vi "Temperature Limit.vi"() -> ()   [LabVIEW 2015]
doc: "This VI simulates the acquisition of temperature, graphs the temperature, and notifies the user if the temperature is over the limit."
panel:
  in  "Start":bool
  in  "Delta t (ms)":i32(slide)=400 scale=50.0..500.0
  in  "Stop":bool
  in  "High Limit":dbl=28.0 format="%.2f"
  out "Temperature":cluster{"Temperature":dbl, "High Limit":dbl}(graph)={"Temperature"=85.88749999999999, "High Limit"=80.0}
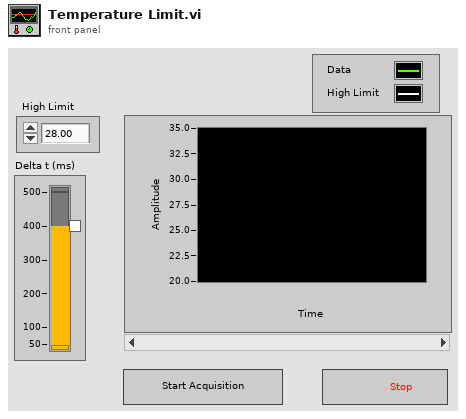
[diagram p1: front panel]
types:
  T1 = enum8{"Enabled", "Disabled", "Disabled and Grayed Out"}
  T2 = enum16{"Always On", "Always Off", "Off While Running"}
  T3 = cluster{"Temperature Value":dbl, "High Limit":dbl}
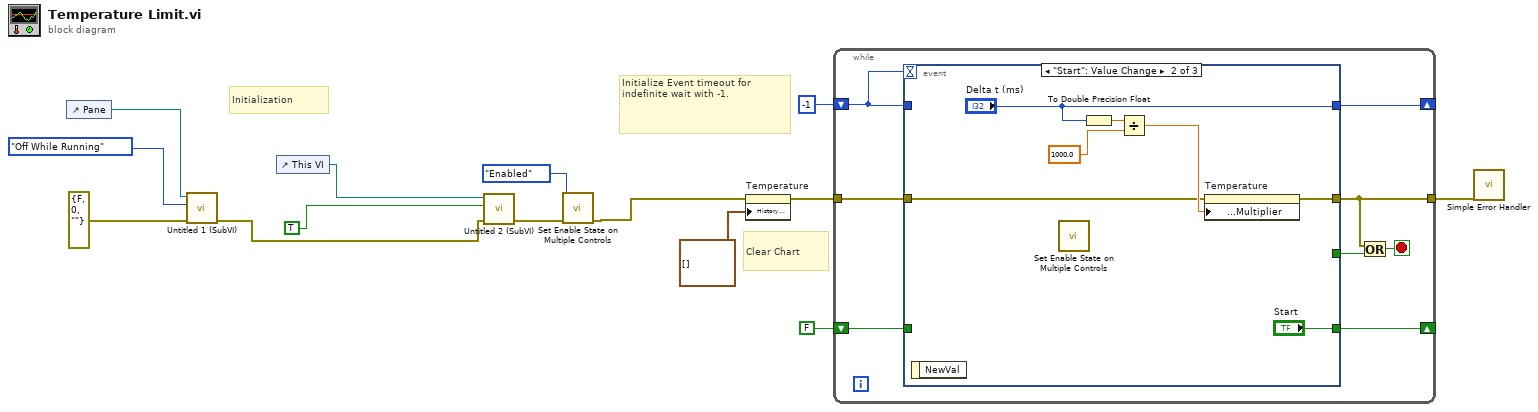
[diagram p0: block diagram]
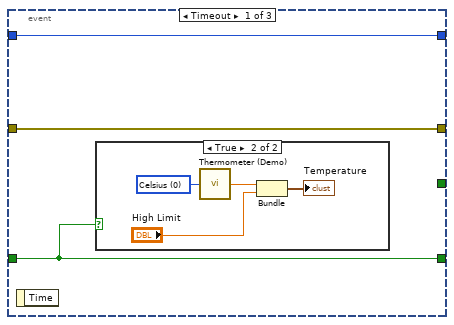
[diagram p2: hidden frame]
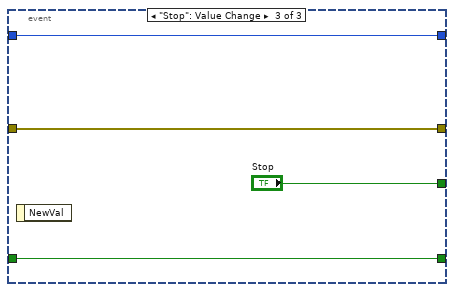
[diagram p4: hidden frame]
diagram:
  # "Clear Chart"
  # "Initialize Event timeout for indefinite wait with -1."
  # "Initialization"
  n1 = control-ref of="Pane"() -> (w5:refnum<vi>)
  n2 = call "Untitled 1 (SubVI).vi"("error in (no error)"=errorcluster {"status"=FALSE, "code"=0, "source"=""}, "Scrollbar Visibility"=T2."Off While Running" ("Horizontal Scrollbar Visibility"), "Pane ref  in"=w5) -> ("error out"=w7:errorcluster)  [unwired: 7 in, 1 out]
  n3 = control-ref of="This VI"() -> (w8:refnum<vi>)
  n4 = call "Untitled 2 (SubVI).vi"("error in (no error)"=w7, "Boolean"=TRUE, "VI in"=w8) -> ("error out"=w3:errorcluster)  [unwired: 7 in, 1 out]
  n5 = call "Set Enable State on Multiple Controls.vi"("Error In"=w3, "Disabled State"=T1."Enabled") -> ("Error Out"=w2:errorcluster)  [unwired: 9 in]
  n6 = property on="Temperature" class="WFChart (strict)"(error in=w2, "History Data"=cluster{"Temperature":dbl, "High Limit":dbl}[] []) -> (error out=w13:errorcluster)  [unwired: 1 in, 1 out]
  n7 = while {
    tunnel: w13 -> [w22]
    tunnel: [w20] -> w11
    shift-right: [w18] -> _
    shift-left: FALSE ("Start") -> [w17]
    shift-right: [w16] -> _
    shift-left: -1 ("Delta t (ms)") -> [w15]
    stop <- w21 stop-if-true
    n8 = event shown="[1] \"Start\": Value Change" {
      selector: _ -> [_ _ _]
      dyn-events: _ -> [_ _ _]
      timeout: w15 -> [_ _ _]
      tunnel: [_ _ "Stop"] -> w19
      tunnel: w22 -> [w25 w30 w39]
      tunnel: [w25 w36 w39] -> w20
      tunnel: [w23 "Start" w38] -> w18
      tunnel: w17 -> [w23 _ w38]
      tunnel: [w24 "Delta t (ms)" w37] -> w16
      tunnel: w15 -> [w24 _ w37]
      event Timeout {
        n9 = event-data() -> ()  [unwired: 1 in, 1 out]
        n10 = case shown="True" w23 {
          frame False {
          }
          frame True {
            w26 = u16 0 items=["Celsius", "Fahrenheit"] ("Units (0: Celsius)")
            n11 = call "Thermometer (Demo).vi"("Units (0: Celsius)"=w26) -> ("Temperature Value"=w27:dbl)
            n12 = Bundle("Temperature Value"=w27, "High Limit"="High Limit") -> (→"Temperature":T3)  [unwired: 1 in]
          }
        }
      }
      event "Start": Value Change {
        n13 = event-data() -> ()  [unwired: 1 in, 1 out]
        n14 = call "Set Enable State on Multiple Controls.vi"() -> ()  [unwired: 11 in, 1 out]
        n15 = To Double Precision Float(number="Delta t (ms)") -> (double precision float=w35:dbl)
        n16 = Divide(x=w35, y=1000.0) -> (x/y=w33:dbl)
        n17 = property on="Temperature" class="WFChart (strict)"(error in=w30, "X Scale.Offset and Multiplier:Multiplier"=w33) -> (error out=w36:errorcluster)  [unwired: 1 in, 1 out]
      }
      event "Stop": Value Change {
        n18 = event-data() -> ()  [unwired: 1 in, 1 out]
      }
    }
    n19 = Or(x=w20, y=w19) -> (x .or. y?=w21:bool)
  }
  n20 = call <vilib>:"Simple Error Handler.vi"("error in (no error)"=w11) -> ()  [unwired: 4 in, 5 out]
